vi "GetObject.vi"(5 "UID":i32, 6 "error in":errorcluster, 9 "VI Interpreter in":refnum<class "VI Interpreter.lvclass">) -> (0 "error out":errorcluster, 1 "found":bool, 3 "VI Interpreter out":refnum<class "VI Interpreter.lvclass">, 4 "value":variant)   [LabVIEW 2014, in "VI Interpreter.lvclass"]
uses:
  VI Interpreter.lvclass
  VI Interpreter.lvclass/VI Interpreter.ctl
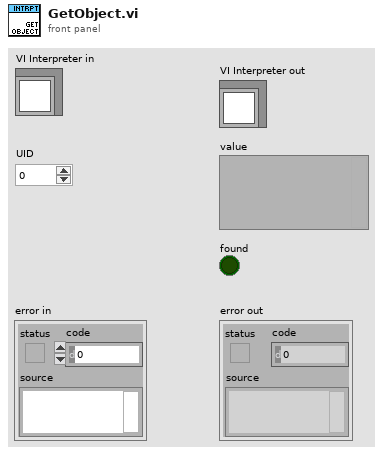
[diagram p1: front panel]
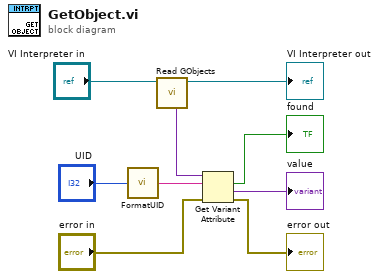
[diagram p0: block diagram]
diagram:
  n1 = call "FormatUID.vi"("UID"="UID") -> ("Name"=w6:string)
  n2 = call "Read GObjects.vi"("VI Interpreter in"="VI Interpreter in") -> ("VI Interpreter out"=→"VI Interpreter out":refnum<class "VI Interpreter.lvclass">, "GObjects"=w8:variant)  [unwired: 7 in]
  n3 = Get Variant Attribute(Variant=w8, name=w6, error in="error in") -> (found=→"found":bool, value=→"value":variant, error out=→"error out":errorcluster)  [unwired: 1 in, 1 out]
